vi "loops_FGV.vi"() -> ()   [LabVIEW 2022 SP3]
panel:
  out "millisecond timer value 2":u32
  out "millisecond timer value":u32
  in  "Set":bool
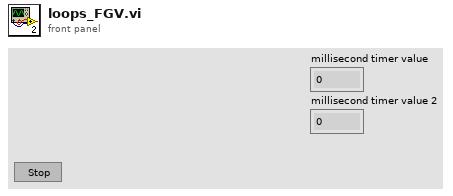
[diagram p1: front panel]
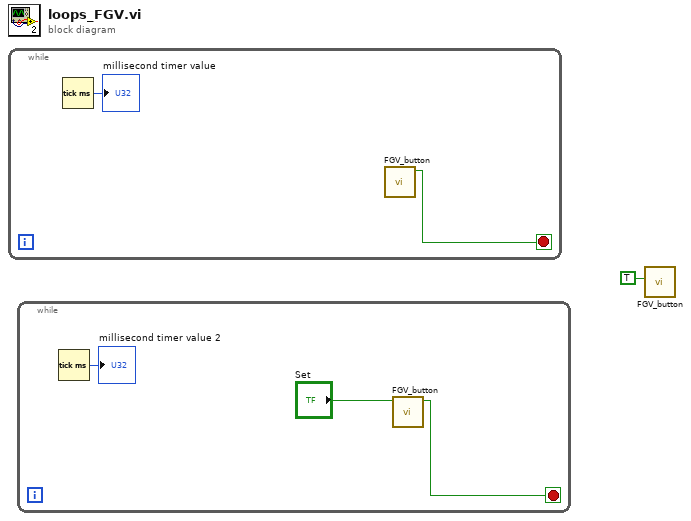
[diagram p0: block diagram]
diagram:
  n1 = while {
    stop <- w3 stop-if-true
    n2 = Tick Count (ms)() -> (millisecond timer value=→"millisecond timer value":u32)
    n3 = call "FGV_button.vi"() -> ("out"=w3:bool)  [unwired: 11 in]
  }
  n4 = while {
    stop <- w6 stop-if-true
    n5 = Tick Count (ms)() -> (millisecond timer value=→"millisecond timer value 2":u32)
    n6 = call "FGV_button.vi"("Set"="Set") -> ("out"=w6:bool)  [unwired: 10 in]
  }
  n7 = call "FGV_button.vi"("Reset"=TRUE) -> ()  [unwired: 10 in, 1 out]
